vi "PC Streaming Host with slow.vi"() -> ()   [LabVIEW 2012]
uses:
  <vilib>/userdefined/High Color/nirio_resource_hc.ctl
  hv cluster control.ctl
  Slow cluster control.ctl
  <vilib>/FPGAPlugInAG/PXI-7951R/niLvFpga_Open_PXI-7951R.vi
  <vilib>/rvi/interface/common/dynamic/niFpgaDynamicAddResources.vi
  <vilib>/Utility/error.llb/Error Cluster From Error Code.vi
  <vilib>/rvi/errors/niLvFpgaAdjustHostInterfaceError.vi
  <vilib>/FPGAPlugInAG/Dynamic/niLvFpga_Close_Dynamic.vi
  <vilib>/rvi/interface/nirviOpenFPGA/nirviOpenFPGA.xnode
  FPGA Bitfiles/ModuDAQ_FPGATarget_TopLevelFPGAw8LE_8T5P+CgHwo4.lvbitx
  <vilib>/rvi/interface/nirviReadWriteControl/nirviReadWriteControl.xnode
  <vilib>/rvi/interface/nirviMethod/nirviMethod.xnode
  <vilib>/rvi/interface/nirviCloseFPGA/nirviCloseFPGA.xnode
  <vilib>/ptbypt/NI_PtbyPt.lvlib
  <vilib>/rvi/interface/Simulation/niFpgaSimulationCallBeginRW.vi
  CAENHVs/CAEN/labview/CAENHVWrapper/CAENHVWrapper.lvlib
  NiFpgaLv.dll
  <vilib>/FPGAPlugInAG/Dynamic/niLvFpga_ReadFifo_Dynamic.vi
  <vilib>/rvi/errors/niLvFpgaMergeErrorWithErrorCode.vi
panel:
  out "fast loop stop":bool
  in  "Channel Cluster":T1={"det_type"=["", "", "", "", "", "", "", ""], "Serial numbers"=["", "", "", "", "", "", "", ""], "Sources"=["", "", "", "", "", "", "", ""], "Trigger level"=[4000, 4000, 4000, 4000, 4000, 4000, 4000, 4000], "Data Record On/Off"=[FALSE, FALSE, FALSE, FALSE, FALSE, FALSE, FALSE, FALSE, TRUE, FALSE, FALSE, FALSE, FALSE, FALSE, FALSE, TRUE], "Number of Channels"=8}
  in  "HV Cluster":T2={"HV Power On/Off"=[TRUE, TRUE], "Set Voltage(V)"=["0", "0", "0", "0", "0", "0", "0", "0"], "HV Tolerance (%)"=1.0, "Current(uA)"=[]}
  out "created path":path
  out "File name":string
  out "Total Data Chunks to Write":dbl
  in  "Tab Control":T3(tab)
  in  "Write mode":bool
  out "directory exists - please wait":u8(slide)
  out "directory ok":bool
  in  "Write Enable":bool
  in  "File Path":path=path "G:/"
  out "File Writing Progress (%)":dbl(slide) scale=0.0..100.0
  in  "Slow Control On":bool
  in  "Fast Data On":bool
  in  "Number of Files to Write":u32=1
  in  "IP Address of NIST Time Server":string(combo)="ntp1.nikhef.nl"
  in  "VISA resource name":refnum<visa-resource-name>="COM8"
  in  "HV Power On/Off":bool[](array[boolean])=[TRUE, TRUE, TRUE, TRUE, TRUE, TRUE, TRUE, TRUE]
  in  "HV Tolerance (%)":dbl=1.0
  out "HV(V)":sgl[](array[numeric])
  in  "IP adress HV2":string="1_0_0"
  in  "IP adress HV1":string="0_0_0"
  out "error HV":errorcluster
  in  "Set Voltage":string[](array[string])=["620", "510", "680", "700", "990", "670", "690", "760"]
  out "Current(uA)":sgl[](array[numeric])
  in  "Current(uA) 2":sgl[](array[numeric])=[107.9, 102.05, 119.4, 122.0, 172.65, 116.8, 120.15, 132.35]
  in  "General Cluster":cluster{"Location":i16}={"Location"=1} {"Location" items=["Purdue", "NIKHEF", "Zurich", "???"]}
  in  "PXI address":T4="RIO0" caption="RIO Device"
  in  "det_type":string[](array[combo])=["NaI(Tl)", "NaI(Tl)", "NaI(Tl)", "NaI(Tl)", "NaI(Tl)", "NaI(Tl)", "NaI(Tl)", "NaI(Tl)"]
  in  "Serial numbers":string[](array[combo])=["SBJ593", "SBJ592", "SBJ590", "SBJ591", "SBJ588", "SBJ589", "SBJ586", "Other"]
  in  "Sources":string[](array[combo])=["Background", "Background", "Ti-44", "Ti-44", "Co-60", "Co-60", "Cs-137", "Cs-137"]
  in  "Trigger level":i16[](array[numeric])=[2000, 2000, 2000, 2000, 2000, 2000, 2000, 2000] caption="Trigger"
  in  "Data Record \nOn/Off":bool[](array[boolean])=[TRUE, TRUE, TRUE, TRUE, TRUE, TRUE, TRUE, TRUE]
  in  "Testpulse Cluster":T5={"Master Pulser On/Off"=FALSE, "Testpulse Turnaround Time (samples)"=14, "Pulse Separation (samples)"=0, "Pulse duration (samples)"=0}
  out "Samples per Data Chunk":u32
  in  "DAQ Info Cluster":T6={"Data Chunks per File"=1000, "Samples per Waveform"=95, "Pretrigger Samples"=15, "circular buffer length (samples)"=1000, "Waveforms per Data Chunk"=5000} {"Waveforms per Data Chunk" format="%.2p"}
  out "Average Throughput":dbl(graph)
  out "Loop Time":u32
  out "Inst. Throughput":dbl format="%#_6p"
  out "Elements in FIFO":u32(graph)
  out "FIFO Overflow":bool
  out "Current Chunk":u32
  out "Current File":i32
  out "Waveform Graph":dynamicdata(graph)
  out "Channel number displayed":i16=-1
  in  "Arduino read \nrate (Hz)":dbl=1.0
  out "Slow time":u64
  out "data":dbl[](array[numeric])
  in  "XON Character":u8=17 format="%.0x"
  in  "XOFF Character":u8=19 format="%.0x"
  out "Slow Cluster":T7
  out "read buffer":string
  out "Bad sensor?":string
  in  "Max Slow Entries per File":i32=86400
  out "Current Slow File":i32
  out "Current Slow Entry":i32
  out "Sensor out of bounds":bool
  out "Temperature":dbl(graph)
  out "Pressure":dbl(graph)
  out "magnetic field y coordinate":dbl(graph)
  out "total magnetic field":dbl(graph)
  out "magnetic field z coordinate":dbl(graph)
  out "magnetic field x coordinate":dbl(graph)
  out "humidity":dbl(graph)
  out "XML String":string
  out "Slow XML":string
  out "error out FAST":errorcluster
  out "error out SLOW":errorcluster
  out "error out XML":errorcluster
  out "NIST Time":u64
  out "NIST Time Failed to Read":bool
  in  "Minutes to wait":u32=5 min=3
  out "UTC format":bool=TRUE
  out "FPGA Timestamp":u64
  out "Time stamp string":string
  out "Stopped":bool
  in  "stop":bool
  # "Channel 0"
  # "Channel 1"
  # "Channel 2"
  # "Channel 3"
  # "Channel 4"
  # "Channel 5"
  # "Channel 6"
  # "Channel 7"
  # "Write continuously"
  # "Write finite number of files"
  # "Program will stop when number of Files to Write is Complete OR if stop is pressed."
  # "These parameters are set by the set_shutdown_HV vi!"
  # "Channel 0"
  # "Channel 1"
  # "Channel 2"
  # "Channel 3"
  # "Channel 4"
  # "Channel 5"
  # "Channel 6"
  # "Channel 7"
  # "This is not a cluster"
  # "Channel 0"
  # "Channel 1"
  # "Channel 2"
  # "Channel 3"
  # "Channel 4"
  # "Channel 5"
  # "Channel 6"
  # "Channel 7"
  # "TODO: Make this look like the \"detectors\" tab"
  # "Waveform/Data Chunk information"
  # "To compare directly on a scope: Horizontal scale: 200 ns/div Vertical scale: ~100 mV/div If 15 pretriggers, delay = 700 ns"
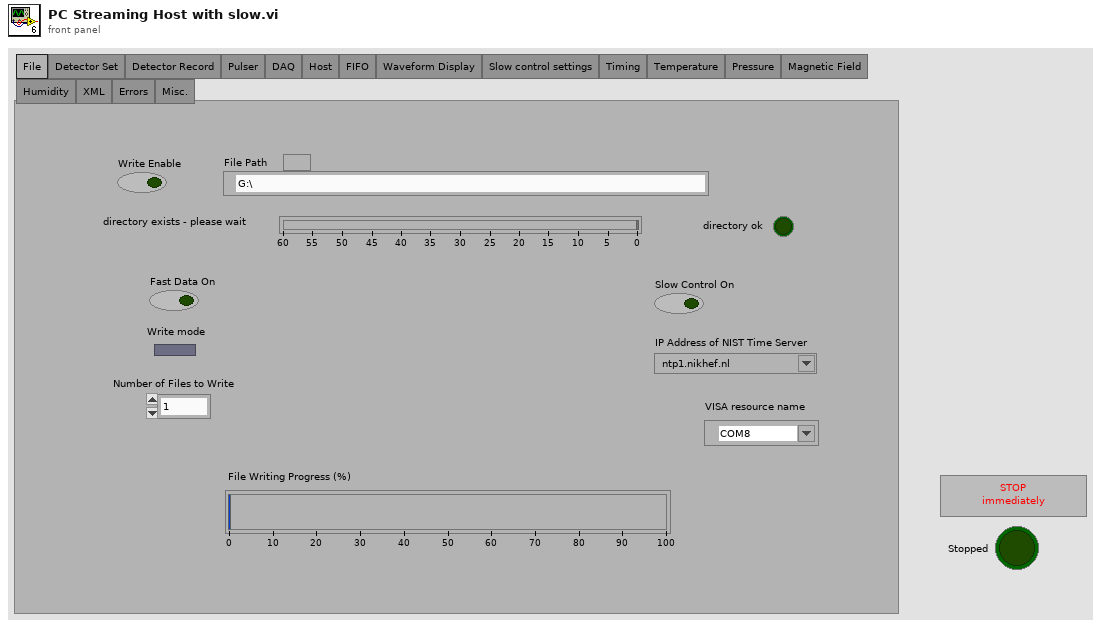
[diagram p1: front panel]
types:
  T1 = cluster{"det_type":string[], "Serial numbers":string[], "Sources":string[], "Trigger level":i16[], "Data Record On/Off":bool[], "Number of Channels":u8}
  T2 = typedef "hv cluster control.ctl" = cluster{"HV Power On/Off":bool[], "Set Voltage(V)":string[], "HV Tolerance (%)":dbl, "Current(uA)":dbl[]}
  T3 = enum32{"File", "Detector Set", "Detector Record", "Pulser", "DAQ", "Host", "FIFO", "Waveform Display", "Slow control settings", "Timing", "Temperature", "Pressure", "Magnetic Field", "Humidity", "XML", "Errors", "Misc."}
  T4 = typedef "nirio_resource_hc.ctl" = tag
  T5 = cluster{"Master Pulser On/Off":bool, "Testpulse Turnaround Time (samples)":u32, "Pulse Separation (samples)":u32, "Pulse duration (samples)":u32}
  T6 = cluster{"Data Chunks per File":u32, "Samples per Waveform":u32, "Pretrigger Samples":u32, "circular buffer length (samples)":u32, "Waveforms per Data Chunk":u32}
  T7 = typedef "Slow cluster control.ctl" = cluster{"Arduino \nParameters":dbl, "Total Number of \nSlow Parameters":i32, "UTC format?":bool, "Sensor Upper \nbounds":i32[], "Sensor Lower \nbounds":i32[], "Descriptions":string[], "datanames":string[]}
  T8 = enum16{"open", "replace", "create", "open or create", "replace or create", "replace or create with confirmation"}
  T9 = enum16{"big-endian, network order", "native, host order", "little-endian"}
  T10 = cluster{"Arduino Parameters":dbl, "Total Number of Slow Parameters":i32, "UTC format?":bool, "Sensor Upper bounds":i32[], "Sensor Lower bounds":i32[], "Descriptions":string[], "datanames":string[]}
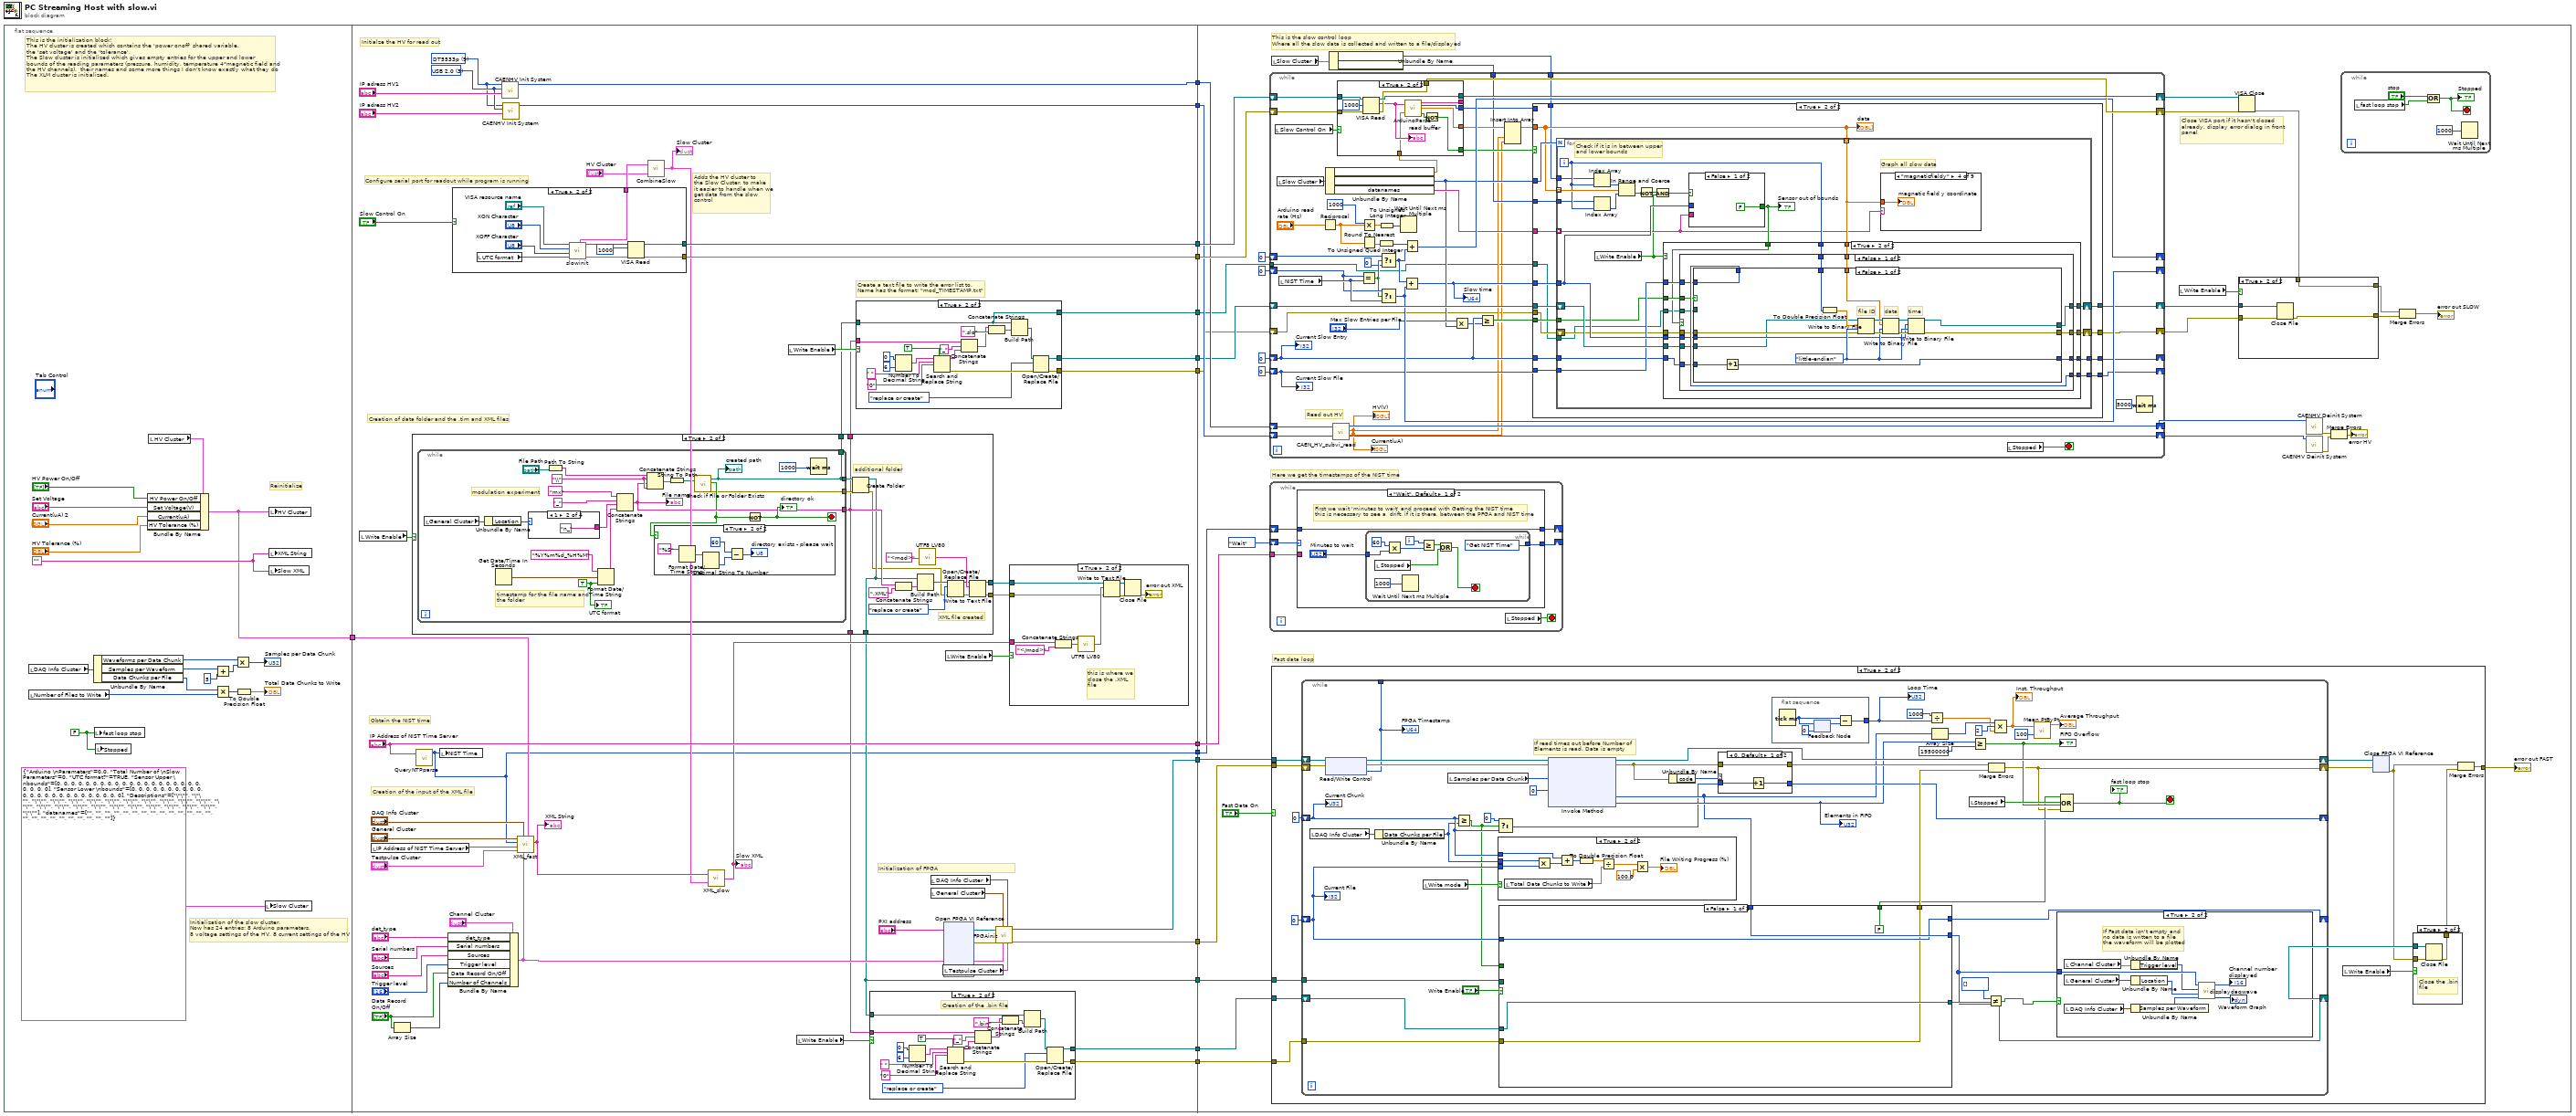
[diagram p0: block diagram]
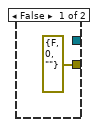
[diagram p2: hidden frame]
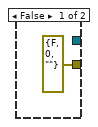
[diagram p3: hidden frame]
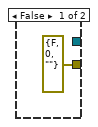
[diagram p6: hidden frame]
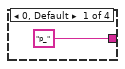
[diagram p7: hidden frame]
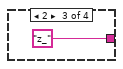
[diagram p8: hidden frame]
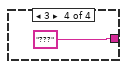
[diagram p9: hidden frame]
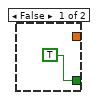
[diagram p11: hidden frame]
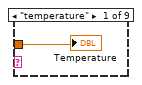
[diagram p13: hidden frame]
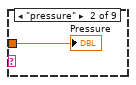
[diagram p14: hidden frame]
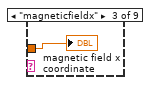
[diagram p15: hidden frame]
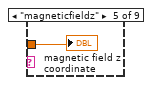
[diagram p16: hidden frame]
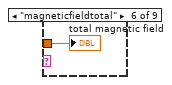
[diagram p17: hidden frame]
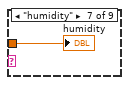
[diagram p18: hidden frame]
diagram:
  n1 = flat-sequence {
    tunnel: [w20] -> w4
    tunnel: ["IP Address of NIST Time Server"] -> w15
    tunnel: [w63] -> w14
    tunnel: [w62] -> w13
    tunnel: [w58] -> w12
    tunnel: [w57] -> w11
    tunnel: [w56] -> w10
    tunnel: [w47] -> w9
    tunnel: [w46] -> w8
    tunnel: [w45] -> w7
    tunnel: [w41] -> w6
    tunnel: [w40] -> w5
    tunnel: w4 -> [w39]
    tunnel: [w38] -> w3
    tunnel: [w37] -> w2
    tunnel: [w36] -> w1
    tunnel: w15 -> [w220]
    tunnel: w14 -> [w212]
    tunnel: w13 -> [w211]
    tunnel: w12 -> [w208]
    tunnel: w11 -> [w210]
    tunnel: w10 -> [w209]
    tunnel: w9 -> [w207]
    tunnel: w8 -> [w206]
    tunnel: w7 -> [w205]
    tunnel: w6 -> [w204]
    tunnel: w5 -> [w203]
    tunnel: w3 -> [w202]
    tunnel: w2 -> [w197]
    tunnel: w1 -> [w194]
    frame #0 {
      w18 = FALSE ("fast loop stop")
      w34 = ""
      # "Initialization of the slow cluster.\nNow has 24 entries: 8 Arduino parameters, \n8 voltage settings of the HV, 8 current settings of the HV"
      # "This is the initialization block!\nThe HV cluster is created which contains the 'power onoff' shared variable, \nthe 'set voltage' and the 'tolerance'.\nThe Slow cluster is initialized which gives empty entries for the upper and lower\nbounds of the reading parameters (pressure, humidity, temperature 4*magnetic field and\nthe HV channels),  their names and some more things I don't know exactly what they do\nThe XLM cluster is initialized."
      # "Reinitialize"
      n2 = local read "DAQ Info Cluster"() -> (w32:T6)
      n3 = local read "Number of Files to Write"() -> (w27:u32)
      n4 = Unbundle By Name(w32) -> ("Waveforms per Data Chunk"=w24:u32, "Samples per Waveform"=w25:u32, "Data Chunks per File"=w26:u32)
      n5 = local write "fast loop stop"(w18) -> ()
      n6 = local write "Stopped"(w18) -> ()
      n7 = local read "HV Cluster"() -> (w33:T2)
      n8 = Bundle By Name(cluster=w33, "HV Power On/Off"="HV Power On/Off", "Set Voltage(V)"="Set Voltage", "Current(uA)"="Current(uA) 2", "HV Tolerance (%)"="HV Tolerance (%)") -> (w20:T2)
      n9 = Add(x=w25, y=u32 5) -> (x+y=w29:u32)
      n10 = Multiply(x=w26, y=w27) -> (x*y=w31:u32)
      n11 = Multiply(x=w24, y=w29) -> (x*y=→"Samples per Data Chunk":u32)
      n12 = To Double Precision Float(number=w31) -> (double precision float=→"Total Data Chunks to Write":dbl)
      n13 = local write "Slow Cluster"(T7 {"Arduino \nParameters"=0.0, "Total Number of \nSlow Parameters"=0, "UTC format?"=TRUE, "Sensor Upper \nbounds"=[0, 0, 0, 0, 0, 0, 0, 0, 0, 0, 0, 0, 0, 0, 0, 0, 0, 0, 0, 0, 0, 0, 0, 0], "Sensor Lower \nbounds"=[0, 0, 0, 0, 0, 0, 0, 0, 0, 0, 0, 0, 0, 0, 0, 0, 0, 0, 0, 0, 0, 0, 0, 0], "Descriptions"=["\"\"", "\"\"", "\"\"", "\"\"", "\"\"", "\"\"", "\"\"", "\"\"", "\"\"", "\"\"", "\"\"", "\"\"", "\"\"", "\"\"", "\"\"", "\"\"", "\"\"", "\"\"", "\"\"", "\"\"", "\"\"", "\"\"", "\"\"", "\"\""], "datanames"=["", "", "", "", "", "", "", "", "", "", "", "", "", "", "", "", "", "", "", "", "", "", "", ""]} ("Slow Cluster 2")) -> ()
      n14 = local write "HV Cluster"(w20) -> ()
      n15 = local write "XML String"(w34) -> ()
      n16 = local write "Slow XML"(w34) -> ()
    }
    frame #1 {
      w65 = 3 items=["TCP/IP"=0, "HS CAENET"=2, "USB 2.0"=3, "CONET Optical Link"=4, "USB VCP"=5] ("LinkType")
      w64 = u32 9 items=["SY1527", "SY2527", "SY4527", "SY5527", "N568", "V65XX", "N1470", "V8100", "", "DT5533p"] ("system")
      # "Obtain the NIST time"
      # "Adds the HV cluster to\nthe Slow Cluster, to make\nit easier to handle when we\nget data from the slow\ncontrol"
      # "Initialization of FPGA"
      # "Initialze the HV for read out"
      # "Create a text file to write the error list to.  \nName has the format: \"mod_TIMESTAMP.txt\""
      # "Creation of the input of the XML file"
      # "Configure serial port for readout while program is running"
      # "Creation of data folder and the .tim and XML files"
      n17 = local read "Write Enable"() -> (w86:bool)
      n18 = local read "IP Address of NIST Time Server"() -> (w77:string)
      n19 = Array Size(array="Data Record \nOn/Off") -> (size(s)=w75:i32)
      n20 = case shown="True" w86 {
        tunnel: [_ w158] -> w59
        tunnel: [_ w150] -> w61
        tunnel: [_ w148] -> w48
        tunnel: [_ w148] -> w42
        tunnel: [_ w147] -> w41
        tunnel: [errorcluster {"status"=FALSE, "code"=0, "source"=""} ("error out") w145] -> w35
        frame False {
        }
        frame True {
          # "XML file created"
          # "additional folder"
          n21 = while {
            tunnel: [w161] -> w159
            tunnel: [w163] -> w160
            tunnel: [w163] -> w158
            tunnel: [w168] -> w148
            stop <- w173 stop-if-true
            w169 = "\\" ("string")
            w176 = TRUE ("UTC format")
            # "modulation experiment"
            # "timestamp for the file name and the folder"
            n22 = local read "General Cluster"() -> (w166:cluster{"Location":i16})
            n23 = Unbundle By Name(w166) -> ("Location"=w165:i16)
            n24 = Get Date/Time In Seconds() -> (seconds since 1Jan1904=w177:timestamp)
            n25 = case shown="1" w165 {
              tunnel: ["p_" ("string") "n_" ("string") "z_" ("string") "???"] -> w167
              frame 0, Default {
              }
              frame 1 {
              }
              frame 2 {
              }
              frame 3 {
              }
            }
            n26 = Path To String(path="File Path") -> (string=w179:string)
            n27 = Format Date/Time String(time format string (%c)="%Y%m%d_%H%M", seconds (now)=w177, UTC format=w176) -> (date/time string=w170:string)
            n28 = Concatenate Strings("mx" ("string"), "_" ("string"), w167, w170) -> (w168:string)
            "File name" <- w168
            n29 = Concatenate Strings(w179, w169, w168, w169) -> (w180:string)
            n30 = String To Path(string=w180) -> (path=w164:path)
            n31 = call <vilib>:"Check if File or Folder Exists.vi"("path"=w164) -> ("error out"=w161:errorcluster, "file or folder exists?"=w162:bool, "dup path"=w163:path)  [unwired: 8 in]
            "created path" <- w163
            n32 = case shown="True" w162 {
              frame False {
              }
              frame True {
                n33 = Format Date/Time String(time format string (%c)="%S") -> (date/time string=w188:string)  [unwired: 2 in]
                n34 = Decimal String To Number(string=w188) -> (number=w186:i32)  [unwired: 2 in, 1 out]
                n35 = Subtract(x=60, y=w186) -> (x-y=→"directory exists - please wait":i32)
              }
            }
            n36 = Not(x=w162) -> (.not. x?=w173:bool)
            "directory ok" <- w173
            n37 = Wait (ms)(milliseconds to wait=1000) -> ()  [unwired: 1 out]
            "UTC format" <- w176
          }
          n38 = Create Folder(path (use dialog)=w160, error in=w159) -> (created path=w147:path, error out=w146:errorcluster)  [unwired: 1 in, 1 out]
          n39 = Concatenate Strings(w148, ".XML" ("substring (\"\")")) -> (w154:string)
          n40 = Build Path(base path=w147, name or relative path=w154) -> (appended path=w153:path)
          n41 = call "UTF8 LV80.vi"("text"="<mod>") -> ("utf-8 text out"=w157:string)
          n42 = Open/Create/Replace File(file path (use dialog)=w153, error in=w146, operation (0:open)=T8."replace or create") -> (refnum out=w156:refnum<file>, error out=w155:errorcluster)  [unwired: 3 in, 1 out]
          n43 = Write to Text File(file (use dialog)=w156, text=w157, error in=w155) -> (refnum out=w150:refnum<file>, error out=w145:errorcluster)  [unwired: 1 in, 1 out]
        }
      }
      n44 = call "QueryNTPparse.vi"("IP Address of NIST Server"="IP Address of NIST Time Server") -> ("NTP Time (server time)"=w38:u64)  [unwired: 1 in, 2 out]
      n45 = local write "NIST Time"(w38) -> ()
      n46 = Bundle By Name(cluster="Channel Cluster", "det_type"="det_type", "Serial numbers"="Serial numbers", "Sources"="Sources", "Trigger level"="Trigger level", "Data Record On/Off"="Data Record \nOn/Off", "Number of Channels"=w75) -> (w44:T1)
      n47 = case shown="True" "Slow Control On" {
        tunnel: [_ w143] -> w63
        tunnel: [_ w142] -> w62
        tunnel: [_ w134] -> w85
        frame False {
        }
        frame True {
          n48 = local read "UTC format"() -> (w137:bool)
          n49 = call "slowinit.vi"("UTC format"=w137, "XOFF Character"="XOFF Character", "XON Character"="XON Character", "VISA resource name"="VISA resource name") -> ("error IO"=w135:errorcluster, "VISA resource name out"=w136:refnum<visa-resource-name>, "Slow Cluster"=w134:T10)  [unwired: 5 in]
          n50 = VISA Read(VISA resource name=w136, byte count=u32 1000, error in (no error)=w135) -> (VISA resource name out=w143:refnum<visa-resource-name>, error out=w142:errorcluster)  [unwired: 2 out]
        }
      }
      n51 = call "CAENHV Init System.vi"("Arg"="IP adress HV1", "LinkType"=w65, "system"=w64) -> ("handle"=w57:i32)  [unwired: 7 in, 1 out]
      n52 = call "CAENHV Init System.vi"("Arg"="IP adress HV2", "LinkType"=w65, "system"=w64) -> ("handle"=w56:i32)  [unwired: 7 in, 1 out]
      n53 = call "XML_fast.vi"("HV Cluster"=w39, "Channel \nCluster"=w44, "DAQ Info Cluster"="DAQ Info Cluster", "Testpulse \nCluster"="Testpulse Cluster", "IP Address of NIST Time Server"=w77, "NIST Time"=w38, "General Cluster"="General Cluster") -> ("XML String"=w80:string)  [unwired: 4 in]
      "XML String" <- w80
      n54 = call "CombineSlow.vi"("HV Cluster"="HV Cluster", "Slow Cluster in"=w85) -> ("Slow Cluster"=w43:T7)
      "Slow Cluster" <- w43
      n55 = call "XML_slow.vi"("Slow Cluster"=w43, "Input String"=w80) -> ("Output String"=w81:string)
      "Slow XML" <- w81
      n56 = local read "Write Enable"() -> (w60:bool)
      n57 = local read "Write Enable"() -> (w49:bool)
      n58 = case shown="True" w60 {
        tunnel: [_ w117] -> w58
        tunnel: w48 -> [_ w109]
        tunnel: w59 -> [_ w108]
        tunnel: [_ w108] -> w40
        tunnel: [errorcluster {"status"=FALSE, "code"=0, "source"=""} ("error out") w107] -> w37
        frame False {
        }
        frame True {
          n59 = Number To Decimal String(number=0, width (-)=i16 6) -> (decimal integer string=w124:string)
          n60 = Search and Replace String(replace all?=TRUE ("replace all? (F)"), input string=w124, search string=" ", replace string="0" ("replace string (\"\")")) -> (result string=w114:string, error out=w119:errorcluster)  [unwired: 4 in, 2 out]
          n61 = Concatenate Strings(w109, "_" ("string"), w114) -> (w112:string)
          n62 = Concatenate Strings(w112, ".slo" ("substring (\"\")")) -> (w116:string)
          n63 = Build Path(base path=w108, name or relative path=w116) -> (appended path=w120:path)
          n64 = Open/Create/Replace File(file path (use dialog)=w120, error in=w119, operation (0:open)=T8."replace or create") -> (refnum out=w117:refnum<file>, error out=w107:errorcluster)  [unwired: 3 in, 1 out]
        }
      }
      n65 = case shown="True" w49 {
        tunnel: [_ w98] -> w47
        tunnel: w42 -> [_ w90]
        tunnel: w41 -> [_ w89]
        tunnel: [errorcluster {"status"=FALSE, "code"=0, "source"=""} ("error out") w88] -> w36
        frame False {
        }
        frame True {
          # "Creation of the .bin file"
          n66 = Number To Decimal String(number=0, width (-)=i16 6) -> (decimal integer string=w105:string)
          n67 = Search and Replace String(replace all?=TRUE ("replace all? (F)"), input string=w105, search string=" ", replace string="0" ("replace string (\"\")")) -> (result string=w95:string, error out=w100:errorcluster)  [unwired: 4 in, 2 out]
          n68 = Concatenate Strings(w90, "_" ("string"), w95) -> (w93:string)
          n69 = Concatenate Strings(w93, ".bin" ("substring (\"\")")) -> (w97:string)
          n70 = Build Path(base path=w89, name or relative path=w97) -> (appended path=w101:path)
          n71 = Open/Create/Replace File(file path (use dialog)=w101, error in=w100, operation (0:open)=T8."replace or create") -> (refnum out=w98:refnum<file>, error out=w88:errorcluster)  [unwired: 3 in, 1 out]
        }
      }
      n72 = local read "DAQ Info Cluster"() -> (w53:T6)
      n73 = local read "General Cluster"() -> (w52:cluster{"Location":i16})
      n74 = local read "Testpulse Cluster"() -> (w51:T5)
      n75 = xnode "Open FPGA VI Reference"("resource name"="PXI address") -> ("FPGA VI Reference Out"=w55:refnum<k20>, "error out"=w54:errorcluster)  [unwired: 1 in]
      n76 = local read "Write Enable"() -> (w68:bool)
      n77 = call "FPGAinit.vi"("Testpulse Cluster"=w51, "DAQ Info Cluster"=w53, "Channel Cluster"=w44, "General Cluster"=w52, "error in"=w54, "FPGA VI Reference In"=w55) -> ("error out"=w45:errorcluster, "FPGA VI Reference Out"=w46:refnum<k20>)  [unwired: 4 in]
      n78 = case shown="True" w68 {
        tunnel: w61 -> [_ w133]
        tunnel: w81 -> [_ w128]
        tunnel: w35 -> [_ w127]
        frame False {
        }
        frame True {
          # "this is where we close the .XML file"
          n79 = Concatenate Strings(w128, "</mod>" ("string")) -> (w129:string)
          n80 = call "UTF8 LV80.vi"("text"=w129) -> ("utf-8 text out"=w132:string)
          n81 = Write to Text File(file (use dialog)=w133, text=w132, error in=w127) -> (refnum out=w131:refnum<file>, error out=w126:errorcluster)  [unwired: 1 in, 1 out]
          n82 = Close File(refnum=w131, error in=w126) -> (error out=→"error out XML":errorcluster)  [unwired: 1 out]
        }
      }
    }
    frame #2 {
      # "This is the slow control loop\nWhere all the slow data is collected and written to a file/displayed"
      # "Fast data loop"
      # "Close VISA port if it hasn't closed already, display error dialog in front panel"
      # "Here we get the timestamps of the NIST time"
      n83 = while {
        shift-right: [w614] -> _
        shift-left: enum16{"Wait", "Get NIST Time", "Write"}."Wait" -> [w615]
        shift-right: [w613] -> _
        shift-left: w202 -> [w612]
        tunnel: w220 -> [w611]
        stop <- w610 stop-if-true
        n84 = case shown="\"Wait\", Default" w615 {
          tunnel: [w618 enum16{"Wait", "Get NIST Time", "Write"}."Wait"] -> w614
          tunnel: [w617 w634] -> w613
          tunnel: w612 -> [w617 w631]
          tunnel: w611 -> [_ w630]
          frame "Wait", Default {
            # "First we wait 'minutes to wait' and proceed with Getting the NIST time\nthis is necessary to see a  drift, if it is there, between the PFGA and NIST time"
            n85 = while {
              tunnel: [enum16{"Wait", "Get NIST Time", "Write"}."Get NIST Time"] -> w618
              tunnel: "Minutes to wait" -> [w620]
              i -> [w623]
              stop <- w624 stop-if-true
              n86 = local read "Stopped"() -> (w622:bool)
              n87 = Multiply(x=60, y=w620) -> (x*y=w619:u32)
              n88 = Wait Until Next ms Multiple(millisecond multiple=u32 1000 ("y")) -> ()  [unwired: 1 out]
              n89 = Greater Or Equal?(x=w623, y=w619) -> (x >= y?=w625:bool)
              n90 = Or(x=w625, y=w622) -> (x .or. y?=w624:bool)
            }
          }
          frame "Get NIST Time" {
            # "Here we get the NIST time"
            n91 = call "QueryNTPparse.vi"("IP Address of NIST Server"=w630) -> ("NTP Time (server time)"=w633:u64, "Time stamp string"=→"Time stamp string":string)  [unwired: 1 in, 1 out]
            "NIST Time" <- w633
            n92 = Equal?(x=w631, y=w633) -> (x = y?=w632:bool)
            "NIST Time Failed to Read" <- w632
            n93 = Select(t=w631, s=w632, f=w633) -> (s? t:f=w634:u64)
          }
        }
        n94 = local read "Stopped"() -> (w610:bool)
      }
      n95 = local read "Slow Cluster"() -> (w224:T7)
      n96 = case shown="True" "Fast Data On" {
        tunnel: w207 -> [_ w450]
        tunnel: w206 -> [_ w449]
        tunnel: w205 -> [w440 w448]
        tunnel: w204 -> [_ w447]
        tunnel: [w440 w442] -> w195
        tunnel: w194 -> [_ w441]
        frame False {
        }
        frame True {
          n97 = while {
            shift-right: [w461] -> w445
            shift-left: w448 -> [w480]
            shift-right: [w487] -> _
            shift-left: u32 0 -> [w484]
            shift-right: [w472] -> _
            shift-left: 0 ("number") -> [w473]
            shift-right: [w488] -> w452
            shift-left: w450 -> [w489]
            tunnel: [w477] -> _
            tunnel: w447 -> [w465]
            shift-right: [w504] -> w446
            shift-left: w449 -> [w467]
            tunnel: w441 -> [w460]
            stop <- w474 stop-if-true
            # "If read times out before Number of Elements is read, Data is empty"
            n98 = local read "DAQ Info Cluster"() -> (w469:T6)
            n99 = xnode "Read/Write Control"("FPGA VI Reference In"=w467, "error in"=w480) -> ("FPGA VI Reference Out"=w479:refnum<k20>, "error out"=w478:errorcluster, "Timestamp"=w477:u64)
            "FPGA Timestamp" <- w477
            n100 = Unbundle By Name(w469) -> ("Data Chunks per File"=w468:u32)
            n101 = local read "Write mode"() -> (w481:bool)
            n102 = local read "Samples per Data Chunk"() -> (w466:u32)
            n103 = Greater Or Equal?(x=w484, y=w468) -> (x >= y?=w462:bool)
            n104 = Select(t=u32 0, s=w462, f=w484) -> (s? t:f=w464:u32)
            n105 = case shown="True" w481 {
              tunnel: w473 -> [_ w523]
              tunnel: w484 -> [_ w521]
              tunnel: w468 -> [_ w514]
              frame False {
              }
              frame True {
                n106 = local read "Total Data Chunks to Write"() -> (w518:dbl)
                n107 = Multiply(x=w514, y=w523) -> (x*y=w522:u32)
                n108 = Add(x=w521, y=w522) -> (x+y=w520:u32)
                n109 = To Double Precision Float(number=w520) -> (double precision float=w519:dbl)
                n110 = Divide(x=w519, y=w518) -> (x/y=w516:dbl)
                n111 = Multiply(x=w516, y=100.0) -> (x*y=→"File Writing Progress (%)":dbl)
              }
            }
            n112 = xnode "Invoke Method"("FPGA VI Reference In"=w479, "error in"=w478, "Number of Elements"=w466, "Timeout (ms)"=0) -> ("FPGA VI Reference Out"=w504:refnum<k20>, "error out"=w501:errorcluster, "Data"=w482:i16[], "Elements Remaining"=w483:u32)
            "Elements in FIFO" <- w483
            n113 = case shown="False" "Write Enable" {
              tunnel: w482 -> [w531 w533]
              tunnel: [w531 _] -> w471
              tunnel: w462 -> [_ w542]
              tunnel: [w528 w541] -> w490
              tunnel: [w532 w540] -> w488
              tunnel: w489 -> [w532 w539]
              tunnel: w473 -> [w530 w538]
              tunnel: [w530 w537] -> w472
              tunnel: [FALSE w536] -> w463
              tunnel: w465 -> [_ w535]
              tunnel: w460 -> [w528 w534]
              frame False {
              }
              frame True {
                n114 = case shown="False" w542 {
                  tunnel: w533 -> [w547 w575]
                  tunnel: [w546 w577] -> w541
                  tunnel: w539 -> [w551 w590]
                  tunnel: [w550 w583] -> w540
                  tunnel: w538 -> [w545 w563]
                  tunnel: [w545 w562] -> w537
                  tunnel: [FALSE w561] -> w536
                  tunnel: w535 -> [_ w564]
                  tunnel: w534 -> [w543 w560]
                  frame False {
                    # "binary writing will write 0 if there is no data"
                    n115 = Not Equal?(x=w547, y=i16[] []) -> (x != y?=w548:bool)
                    n116 = case shown="True" w548 {
                      tunnel: w551 -> [w553 w559]
                      tunnel: [w553 w558] -> w550
                      tunnel: [w552 w557] -> w546
                      tunnel: w547 -> [_ w555]
                      tunnel: w543 -> [w552 w554]
                      frame False {
                      }
                      frame True {
                        n117 = Write to Binary File(file (use dialog)=w559, data=w555, error in=w554, 9:T9."little-endian" ("byte order (0:big-endian, network order)")) -> (refnum out=w558:refnum<file>, error out=w557:errorcluster)  [unwired: 2 in, 1 out]
                      }
                    }
                  }
                  frame True {
                    # "little-endian is windows and linux way of writing and reading binary not the standard in labview !?!"
                    # "opening the new ones"
                    # "closing files"
                    n118 = Increment(x=w563) -> (x+1=w562:i32)
                    n119 = Number To Decimal String(number=w562, width (-)=i16 6) -> (decimal integer string=w592:string)
                    n120 = Close File(refnum=w590, error in=w560) -> (error out=w589:errorcluster)  [unwired: 1 out]
                    n121 = local read "File name"() -> (w571:string)
                    n122 = Search and Replace String(replace all?=TRUE ("replace all? (F)"), input string=w592, search string=" ", replace string="0" ("replace string (\"\")"), error in=w589) -> (result string=w582:string, error out=w588:errorcluster)  [unwired: 3 in, 2 out]
                    n123 = Concatenate Strings(w571, "_" ("string"), w582) -> (w578:string)
                    n124 = local read "Samples per Data Chunk"() -> (w570:u32)
                    n125 = Concatenate Strings(w578, ".bin" ("substring (\"\")")) -> (w580:string)
                    n126 = Equal?(x="Write mode", y=TRUE) -> (x = y?=w569:bool)
                    n127 = Equal?(x="Number of Files to Write", y=w562) -> (x = y?=w568:bool)
                    n128 = And(x=w568, y=w569) -> (x .and. y?=w561:bool)
                    n129 = Build Path(base path=w564, name or relative path=w580) -> (appended path=w587:path)
                    n130 = Open/Create/Replace File(file path (use dialog)=w587, error in=w588, operation (0:open)=T8."replace or create") -> (refnum out=w584:refnum<file>, error out=w585:errorcluster)  [unwired: 3 in, 1 out]
                    n131 = Array Size(array=w575) -> (size(s)=w574:i32)
                    n132 = Equal?(x=w574, y=w570) -> (x = y?=w573:bool)
                    n133 = Not Equal?(x=w575, y=i16[] []) -> (x != y?=w576:bool)
                    n134 = And(x=w576, y=w573) -> (x .and. y?=w572:bool)
                    n135 = case shown="True" w572 {
                      tunnel: w585 -> [w597 w604]
                      tunnel: w584 -> [w598 w603]
                      tunnel: [w598 w602] -> w583
                      tunnel: [w597 w601] -> w577
                      tunnel: w575 -> [_ w600]
                      frame False {
                      }
                      frame True {
                        n136 = Write to Binary File(file (use dialog)=w603, data=w600, error in=w604, 9:T9."little-endian" ("byte order (0:big-endian, network order)")) -> (refnum out=w602:refnum<file>, error out=w601:errorcluster)  [unwired: 2 in, 1 out]
                      }
                    }
                  }
                }
              }
            }
            n137 = Unbundle By Name(w501) -> ("code"=w502:i32)
            n138 = case shown="0, Default" w502 {
              tunnel: [w607 errorcluster {"status"=FALSE, "code"=0, "source"=""} ("error constant")] -> w491
              tunnel: w501 -> [w607 _]
              tunnel: w464 -> [w606 w608]
              tunnel: [w605 w608] -> w487
              frame 0, Default {
                n139 = Increment(x=w606) -> (x+1=w605:u32)
              }
              frame -50400 {
                # "Timeout"
              }
            }
            n140 = flat-sequence {
              tunnel: [w527] -> w495
              frame #0 {
                n141 = Tick Count (ms)() -> (millisecond timer value=w526:u32)
                n142 = feedback #1(u32 0 ("millisecond timer value")) -> (w525:u32)
                n143 = feedback-in #1(w526) -> ()
                n144 = Subtract(x=w526, y=w525) -> (x-y=w527:u32)
              }
            }
            n145 = Divide(x=u32 1000, y=w495) -> (x/y=w497:dbl)
            n146 = Array Size(array=w482) -> (size(s)=w500:i32)
            n147 = local read "Stopped"() -> (w476:bool)
            n148 = Greater Or Equal?(x=w483, y=u32 19500000) -> (x >= y?=w475:bool)
            "FIFO Overflow" <- w475
            n149 = Not Equal?(x=i16[] [], y=w471) -> (x != y?=w459:bool)
            n150 = Merge Errors(w491, w490) -> (w461:errorcluster)
            n151 = Compound Arithmetic op=MULTIPLY(w500, 2 ("y"), w497) -> (w494:dbl)
            "Inst. Throughput" <- w494
            n152 = call <vilib>:"Mean PtByPt.vi"("x"=w494, "sample length"=100) -> ("mean"=→"Average Throughput":dbl)  [unwired: 2 in, 1 out]
            n153 = case shown="True" w459 {
              tunnel: w471 -> [_ w513]
              frame False {
              }
              frame True {
                # "If Fast data isn't empty and\nno data is written to a file\nthe waveform will be plotted"
                n154 = local read "Channel Cluster"() -> (w511:T1)
                n155 = local read "General Cluster"() -> (w509:cluster{"Location":i16})
                n156 = local read "DAQ Info Cluster"() -> (w507:T6)
                n157 = Unbundle By Name(w511) -> ("Trigger level"=w510:i16[])
                n158 = Unbundle By Name(w509) -> ("Location"=w508:i16)
                n159 = Unbundle By Name(w507) -> ("Samples per Waveform"=w506:u32)
                n160 = call "displaydaqwave.vi"("Samples per Waveform"=w506, "Location"=w508, "Trigger level"=w510, "Waveform from DAQ"=w513) -> ("Waveform Graph"=→"Waveform Graph":dynamicdata, "Channel number displayed"=→"Channel number displayed":i16)  [unwired: 6 in]
              }
            }
            n161 = Compound Arithmetic op=OR(w463, w476, w475, w461) -> (w474:bool)
            "fast loop stop" <- w474
            "Loop Time" <- w495
            "Current Chunk" <- w484
            "Current File" <- w473
          }
          n162 = local read "Write Enable"() -> (w454:bool)
          n163 = xnode "Close FPGA VI Reference"("FPGA VI Reference In"=w446, "error in"=w445) -> ("error out"=w444:errorcluster)
          n164 = case shown="True" w454 {
            tunnel: w444 -> [w455 w457]
            tunnel: w452 -> [_ w458]
            tunnel: [w455 w456] -> w443
            frame False {
            }
            frame True {
              # "Close the .bin\nfile"
              n165 = Close File(refnum=w458, error in=w457) -> (error out=w456:errorcluster)  [unwired: 1 out]
            }
          }
          n166 = Merge Errors(w444, w443) -> (w442:errorcluster)
        }
      }
      "error out FAST" <- w195
      n167 = Unbundle By Name(w224) -> ("Sensor Upper \nbounds"=w214:i32[], "Sensor Lower \nbounds"=w213:i32[])
      n168 = while {
        shift-right: [w270] -> _
        shift-left: u64 0 -> [w274]
        shift-right: [w267] -> _
        shift-left: u64 0 -> [w272]
        shift-right: [w253] -> w219
        shift-left: w208 -> [w276]
        shift-right: [w249] -> _
        shift-left: 0 -> [w250]
        shift-right: [w248] -> _
        shift-left: 0 -> [w252]
        tunnel: w214 -> [w242]
        tunnel: w213 -> [w241]
        tunnel: w203 -> [w232]
        shift-right: [w278] -> w216
        shift-left: w212 -> [w240]
        shift-right: [w277] -> w215
        shift-left: w211 -> [w239]
        shift-right: [w236] -> w218
        shift-left: w210 -> [w238]
        shift-right: [w234] -> w217
        shift-left: w209 -> [w237]
        shift-right: [w229] -> w196
        shift-left: w197 -> [w230]
        stop <- w233 stop-if-true
        # "Read out HV"
        n169 = local read "Slow Control On"() -> (w256:bool)
        n170 = local read "Slow Cluster"() -> (w261:T7)
        n171 = local read "NIST Time"() -> (w275:u64)
        n172 = Reciprocal(x="Arduino read \nrate (Hz)") -> (1/x=w264:dbl)
        n173 = Unbundle By Name(w261) -> ("Arduino \nParameters"=w257:dbl, "Total Number of \nSlow Parameters"=w246:i32, "datanames"=w254:string[])
        n174 = call "CAEN_HV_subvi_read.vi"("handle HV1"=w238, "handle HV2"=w237) -> ("handle HV1 out"=w236:i32, "HV"=w235:sgl[], "Current"=w231:sgl[], "handle HV2 out"=w234:i32)  [unwired: 1 in, 1 out]
        "HV(V)" <- w235
        "Current(uA)" <- w231
        n175 = case shown="True" w256 {
          tunnel: [_ w290] -> w278
          tunnel: [_ w289] -> w277
          tunnel: [_ w287] -> w260
          tunnel: [_ w286] -> _
          tunnel: [TRUE w282] -> w255
          tunnel: [_ w284] -> w259
          tunnel: w257 -> [_ w283]
          tunnel: w240 -> [_ w281]
          tunnel: w239 -> [_ w280]
          frame False {
          }
          frame True {
            n176 = VISA Read(VISA resource name=w281, byte count=u32 1000, error in (no error)=w280) -> (VISA resource name out=w290:refnum<visa-resource-name>, read buffer=w288:string, error out=w289:errorcluster)  [unwired: 1 out]
            "read buffer" <- w288
            n177 = call "ArduinoParse.vi"("read buffer"=w288, "Expected Arduino Parameters"=w283) -> ("Number Arduino Parameters"=w287:i32, "Arduino Data Names"=w286:string[], "Arduino Data"=w284:dbl[], "Arduino Read Failed?"=w285:bool)
            n178 = Not(x=w285) -> (.not. x?=w282:bool)
          }
        }
        n179 = Equal?(x=w274, y=w275) -> (x = y?=w273:bool)
        n180 = Multiply(x=u32 1000 ("millisecond multiple"), y=w264) -> (x*y=w266:dbl)
        n181 = Round To Nearest(number=w264) -> (nearest integer value=w263:dbl)
        n182 = To Unsigned Quad Integer(1:w263) -> (0:w262:u64)
        n183 = To Unsigned Long Integer(number=w266) -> (unsigned 32bit integer=w265:u32)
        n184 = Select(t=w272, s=w273, f=0) -> (s? t:f=w268:u64)
        n185 = Select(t=w274, s=w273, f=w275) -> (s? t:f=w270:u64)
        n186 = Wait Until Next ms Multiple(millisecond multiple=w265) -> ()  [unwired: 1 out]
        n187 = Add(x=w268, y=w270) -> (x+y=w243:u64)
        "Slow time" <- w243
        n188 = Add(x=w262, y=w268) -> (x+y=w267:u64)
        n189 = Multiply(x="Max Slow Entries per File", y=w246) -> (x*y=w245:i32)
        n190 = Greater Or Equal?(x=w250, y=w245) -> (x >= y?=w251:bool)
        n191 = Insert Into Array(array=w259, new element #1=w235, new element #2=w231) -> (w258:dbl[])  [unwired: 1 in]
        n192 = case shown="True" w255 {
          tunnel: w276 -> [w295 w311]
          tunnel: w243 -> [_ w310]
          tunnel: [w295 w307] -> w253
          tunnel: w260 -> [_ _]
          tunnel: w258 -> [_ w301]
          tunnel: w254 -> [_ w309]
          tunnel: w246 -> [_ w308]
          tunnel: w252 -> [w293 w306]
          tunnel: w251 -> [_ w305]
          tunnel: w250 -> [w294 w304]
          tunnel: [w294 w303] -> w249
          tunnel: [w293 w302] -> w248
          tunnel: w242 -> [_ w300]
          tunnel: w241 -> [_ w299]
          tunnel: w232 -> [_ w296]
          tunnel: w230 -> [w292 w298]
          tunnel: [w292 w297] -> w229
          frame False {
          }
          frame True {
            n193 = for {
              N: w308 -> [_]
              tunnel: w310 -> [w332]
              tunnel: w301 -> [w334] mode=indexing
              tunnel: w309 -> [w320] mode=indexing
              tunnel: w301 -> [w321] mode=indexing
              tunnel: w306 -> [w329]
              tunnel: w305 -> [w327]
              tunnel: w304 -> [w326]
              tunnel: [w325] -> w303
              tunnel: [w324] -> w302
              shift-right: [w330] -> w307
              shift-left: w311 -> [w331]
              tunnel: w300 -> [w319]
              tunnel: w299 -> [w318]
              shift-right: [w315] -> w297
              shift-left: w298 -> [w314]
              tunnel: w296 -> [w313]
              i -> [w328]
              # "Check if it is in between upper \nand lower bounds"
              # "Graph all slow data"
              n194 = Index Array(array=w319, index=w328) -> (element=w316:i32)
              n195 = Index Array(array=w318, index=w328) -> (element=w317:i32)
              n196 = local read "Write Enable"() -> (w312:bool)
              n197 = In Range and Coerce(upper limit=w316, x=w334, lower limit=w317) -> (In Range?=w323:bool)  [unwired: 1 out]
              n198 = Not(x=w323) -> (.not. x?=w335:bool)
              n199 = And(x=w335, y=w312) -> (x .and. y?=w333:bool)
              n200 = case shown="False" w333 {
                tunnel: w320 -> [_ w428]
                tunnel: w332 -> [_ _]
                tunnel: [FALSE ("Sensor out of bounds") TRUE ("Sensor out of bounds")] -> w322
                frame False {
                }
                frame True {
                  "Bad sensor?" <- w428
                }
              }
              "Sensor out of bounds" <- w322
              n201 = case shown="True" w312 {
                tunnel: [w344 w360] -> w324
                tunnel: w321 -> [_ w359]
                tunnel: w332 -> [_ w358]
                tunnel: w331 -> [w346 w357]
                tunnel: [w346 w356] -> w330
                tunnel: w329 -> [w344 w355]
                tunnel: w328 -> [_ w354]
                tunnel: w327 -> [_ w353]
                tunnel: w326 -> [w345 w352]
                tunnel: [w345 w351] -> w325
                tunnel: w322 -> [_ w350]
                tunnel: w313 -> [_ w349]
                tunnel: [w343 w348] -> w315
                tunnel: w314 -> [w343 w347]
                frame False {
                }
                frame True {
                  n202 = case shown="False" w350 {
                    tunnel: [w373 w425] -> w360
                    tunnel: w359 -> [w372 _]
                    tunnel: w358 -> [w371 _]
                    tunnel: w357 -> [w370 w424]
                    tunnel: [w369 w424] -> w356
                    tunnel: w355 -> [w368 w425]
                    tunnel: w354 -> [w367 _]
                    tunnel: w353 -> [w366 _]
                    tunnel: w352 -> [w365 w426]
                    tunnel: [w364 w426] -> w351
                    tunnel: w349 -> [w363 _]
                    tunnel: [w362 w423] -> w348
                    tunnel: w347 -> [w361 w423]
                    frame False {
                      n203 = case shown="False" w366 {
                        tunnel: [w381 w395] -> w373
                        tunnel: w372 -> [w383 w403]
                        tunnel: w371 -> [w382 w402]
                        tunnel: w370 -> [w375 w401]
                        tunnel: [w377 w399] -> w369
                        tunnel: w368 -> [w381 w398]
                        tunnel: w367 -> [w380 w397]
                        tunnel: w365 -> [w379 _]
                        tunnel: [w378 0] -> w364
                        tunnel: w363 -> [_ w393]
                        tunnel: [w374 w391] -> w362
                        tunnel: w361 -> [w376 w392]
                        frame False {
                          w384 = T9."little-endian" ("byte order (0:big-endian, network order)")
                          # "time"
                          # "data"
                          # "file ID"
                          n204 = Increment(x=w379) -> (x+1=w378:i32)
                          n205 = To Double Precision Float(number=w380) -> (double precision float=w385:dbl)
                          n206 = Write to Binary File(file (use dialog)=w375, data=w385, error in=w376, 9:w384) -> (refnum out=w388:refnum<file>, error out=w389:errorcluster)  [unwired: 2 in, 1 out]
                          n207 = Write to Binary File(file (use dialog)=w388, data=w383, error in=w389, 9:w384) -> (refnum out=w387:refnum<file>, error out=w386:errorcluster)  [unwired: 2 in, 1 out]
                          n208 = Write to Binary File(file (use dialog)=w387, data=w382, error in=w386, 9:w384) -> (refnum out=w377:refnum<file>, error out=w374:errorcluster)  [unwired: 2 in, 1 out]
                        }
                        frame True {
                          w404 = T9."little-endian" ("byte order (0:big-endian, network order)")
                          w394 = TRUE ("replace all? (F)")
                          # "time"
                          # "data"
                          # "file ID"
                          # "opening the new ones"
                          # "closing files"
                          n209 = Increment(x=w398) -> (x+1=w395:i32)
                          n210 = Number To Decimal String(number=w395, width (-)=i16 6) -> (decimal integer string=w419:string)
                          n211 = Close File(refnum=w401, error in=w392) -> (error out=w417:errorcluster)  [unwired: 1 out]
                          n212 = local read "File name"() -> (w410:string)
                          n213 = Search and Replace String(replace all?=w394, case sensitive?=w394, input string=w419, search string=" ", replace string="0" ("replace string (\"\")"), error in=w417) -> (result string=w414:string, error out=w416:errorcluster)  [unwired: 2 in, 2 out]
                          n214 = Concatenate Strings(w410, "_" ("string"), w414) -> (w411:string)
                          n215 = Concatenate Strings(w411, ".slo" ("substring (\"\")")) -> (w412:string)
                          n216 = Build Path(base path=w393, name or relative path=w412) -> (appended path=w390:path)
                          n217 = Open/Create/Replace File(file path (use dialog)=w390, error in=w416, operation (0:open)=T8."replace or create") -> (refnum out=w400:refnum<file>)  [unwired: 3 in, 2 out]
                          n218 = To Double Precision Float(number=w397) -> (double precision float=w405:dbl)
                          n219 = Write to Binary File(file (use dialog)=w400, data=w405, 9:w404) -> (refnum out=w408:refnum<file>, error out=w409:errorcluster)  [unwired: 3 in, 1 out]
                          n220 = Write to Binary File(file (use dialog)=w408, data=w403, error in=w409, 9:w404) -> (refnum out=w407:refnum<file>, error out=w406:errorcluster)  [unwired: 2 in, 1 out]
                          n221 = Write to Binary File(file (use dialog)=w407, data=w402, error in=w406, 9:w404) -> (refnum out=w399:refnum<file>, error out=w391:errorcluster)  [unwired: 2 in, 1 out]
                        }
                      }
                    }
                    frame True {
                    }
                  }
                }
              }
              n222 = case shown="\"magneticfieldy\"" w320 {
                tunnel: w321 -> [w336 w337 w338 w339 w340 w341 w342 _ _]
                frame "temperature" {
                  "Temperature" <- w336
                }
                frame "pressure" {
                  "Pressure" <- w337
                }
                frame "magneticfieldx" {
                  "magnetic field x coordinate" <- w338
                }
                frame "magneticfieldy" {
                  "magnetic field y coordinate" <- w339
                }
                frame "magneticfieldz" {
                  "magnetic field z coordinate" <- w340
                }
                frame "magneticfieldtotal" {
                  "total magnetic field" <- w341
                }
                frame "humidity" {
                  "humidity" <- w342
                }
                frame "seconds" {
                }
                frame "", Default {
                }
              }
            }
            "data" <- w301
          }
        }
        n223 = local read "Stopped"() -> (w233:bool)
        n224 = Wait (ms)(milliseconds to wait=u32 5000) -> ()  [unwired: 1 out]
        "Current Slow Entry" <- w250
        "Current Slow File" <- w252
      }
      n225 = local read "Write Enable"() -> (w225:bool)
      n226 = VISA Close(VISA resource name=w216, error in (no error)=w215) -> (error out=w193:errorcluster)
      n227 = case shown="True" w225 {
        tunnel: w219 -> [_ w435]
        tunnel: w196 -> [w430 w434]
        tunnel: w193 -> [w431 w432]
        tunnel: [w430 w433] -> w192
        tunnel: [w431 w432] -> w191
        frame False {
        }
        frame True {
          n228 = Close File(refnum=w435, error in=w434) -> (error out=w433:errorcluster)  [unwired: 1 out]
        }
      }
      n229 = call "CAENHV Deinit System.vi"("handle"=w218) -> ("error out"=w223:errorcluster)  [unwired: 10 in]
      n230 = call "CAENHV Deinit System.vi"("handle"=w217) -> ("error out"=w222:errorcluster)  [unwired: 10 in]
      n231 = Merge Errors(w223, w222) -> (→"error HV":errorcluster)
      n232 = while {
        stop <- w437 stop-if-true
        n233 = local read "fast loop stop"() -> (w436:bool)
        n234 = Compound Arithmetic op=OR("stop", w436) -> (w437:bool)
        "Stopped" <- w437
        n235 = Wait Until Next ms Multiple(millisecond multiple=u32 1000 ("y")) -> ()  [unwired: 1 out]
      }
      n236 = Merge Errors(w191, w192) -> (→"error out SLOW":errorcluster)
    }
  }
